vi "Receive-graph.vi"() -> ()   [LabVIEW 2020]
panel:
  out "Numeric":dbl
  out "return count":u32
  in  "byte count":u32
  in  "VISA resource name":refnum<visa-resource-name>
  in  "?":bool
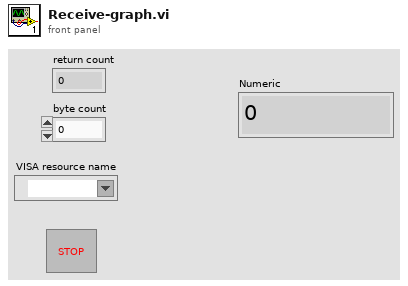
[diagram p1: front panel]
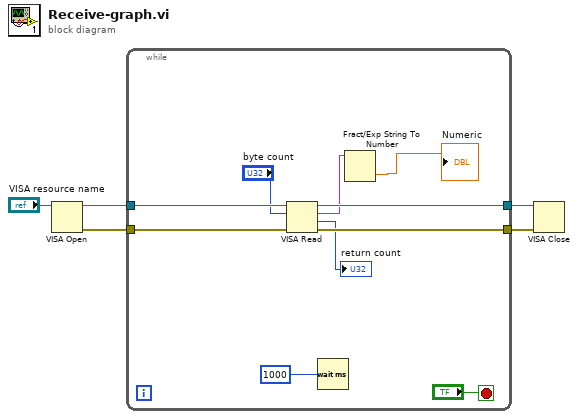
[diagram p0: block diagram]
diagram:
  n1 = VISA Open(VISA resource name="VISA resource name") -> (VISA resource name=w5:refnum<visa-resource-name>, error out=w4:errorcluster)  [unwired: 4 in]
  n2 = while {
    tunnel: w5 -> [w13]
    tunnel: w4 -> [w12]
    tunnel: [w11] -> w3
    tunnel: [w10] -> w2
    stop <- "?" stop-if-true
    n3 = VISA Read(VISA resource name=w13, byte count="byte count", error in (no error)=w12) -> (VISA resource name out=w10:refnum<visa-resource-name>, read buffer=w8:string, return count=→"return count":u32, error out=w11:errorcluster)
    n4 = Wait (ms)(milliseconds to wait=u32 1000) -> ()  [unwired: 1 out]
    n5 = Fract/Exp String To Number(string=w8) -> (number=→"Numeric":dbl)  [unwired: 3 in, 1 out]
  }
  n6 = VISA Close(VISA resource name=w2, error in (no error)=w3) -> ()  [unwired: 1 out]
